vi "Next Identity.vi"(5 "Username":string, 6 "Password":string, 7 "Address":string, 8 "Error In":errorcluster) -> (0 "Error Out":errorcluster)   [LabVIEW 2018, in "Tests.lvlib" / "Agent.lvlib"]
uses:
  Agent.lvlib
  <vilib>/addons/_JKI Toolkits/Caraya/classes/Test/Test.lvclass
  <vilib>/addons/_JKI Toolkits/Caraya/classes/Assert/Assert.lvclass
  src/Toolkit/Agent/Agent.lvclass
  src/Toolkit/Agent Identity/Agent Identity.lvclass
  src/Toolkit/Agent Identity/Support/Create from Agent.vi
  src/Toolkit/Agent/Typedefs/Results.ctl
  src/Toolkit/Agent Identity/Support/Destroy to Agent.vi
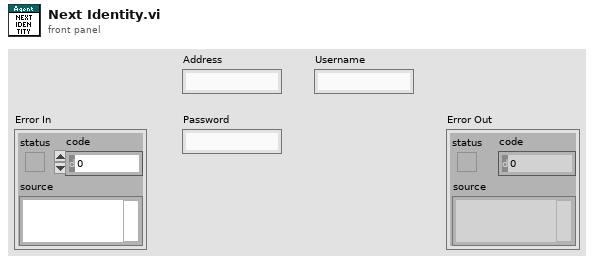
[diagram p1: front panel]
types:
  T1 = typedef "Toolkit.lvlib/Agent.lvclass/Results.ctl" = enum32{"Success", "End of Identities"}
  T2 = typedef "Toolkit.lvlib/Agent.lvclass/Results.ctl" = i32
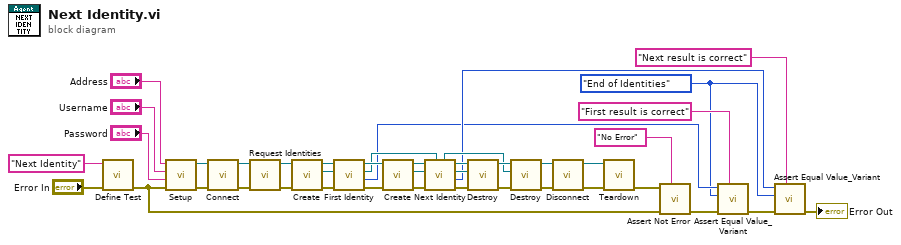
[diagram p0: block diagram]
diagram:
  w1 = Results."End of Identities" ("Result")
  n1 = call <vilib>:"Define Test.vi"("error in (no error)"="Error In", "Label (VI Title)"="Next Identity") -> ("error out"=w36:errorcluster)  [unwired: 9 in]
  n2 = call "Setup.vi"("Error In"=w36, "Password"="Password", "Username"="Username", "Address"="Address") -> ("Error Out"=w34:errorcluster, "Agent"=w35:refnum<class "Agent.lvclass">)  [unwired: 6 in]
  n3 = call "Connect.vi"("Error In"=w34, "Agent In"=w35) -> ("Error Out"=w32:errorcluster, "Agent Out"=w33:refnum<class "Agent.lvclass">)  [unwired: 8 in]
  n4 = call "Request Identities.vi"("Error In"=w32, "Agent In"=w33) -> ("Error Out"=w30:errorcluster, "Agent Out"=w31:refnum<class "Agent.lvclass">)  [unwired: 8 in]
  n5 = call-poly "Create.vi"("Error In"=w30, "Agent In"=w31) -> ("Error Out"=w28:errorcluster, "Identity"=w27:refnum<class "Agent Identity.lvclass">, "Agent Out"=w29:refnum<class "Agent.lvclass">)  [unwired: 7 in]
  n6 = call "First Identity.vi"("Error In"=w28, "Identity In"=w27, "Agent In"=w29) -> ("Error Out"=w17:errorcluster, "Result"=w2:T2, "Identity Out"=w8:refnum<class "Agent Identity.lvclass">, "Agent Out"=w18:refnum<class "Agent.lvclass">)  [unwired: 5 in]
  n7 = call-poly "Create.vi"("Error In"=w17, "Agent In"=w18) -> ("Error Out"=w14:errorcluster, "Identity"=w10:refnum<class "Agent Identity.lvclass">, "Agent Out"=w13:refnum<class "Agent.lvclass">)  [unwired: 7 in]
  n8 = call "Next Identity.vi"("Previous In"=w8, "Error In"=w14, "Next In"=w10, "Agent In"=w13) -> ("Error Out"=w11:errorcluster, "Result"=w6:T2, "Next Out"=w9:refnum<class "Agent Identity.lvclass">, "Agent Out"=w12:refnum<class "Agent.lvclass">, "Previous Out"=w7:refnum<class "Agent Identity.lvclass">)  [unwired: 3 in]
  n9 = call-poly "Destroy.vi"("Error In"=w11, "Identity"=w9, "Agent In"=w12) -> ("Error Out"=w15:errorcluster, "Agent Out"=w16:refnum<class "Agent.lvclass">)  [unwired: 7 in]
  n10 = call-poly "Destroy.vi"("Error In"=w15, "Identity"=w7, "Agent In"=w16) -> ("Error Out"=w24:errorcluster, "Agent Out"=w25:refnum<class "Agent.lvclass">)  [unwired: 7 in]
  n11 = call "Disconnect.vi"("Error In"=w24, "Agent In"=w25) -> ("Error Out"=w23:errorcluster, "Agent Out"=w22:refnum<class "Agent.lvclass">)  [unwired: 8 in]
  n12 = call "Teardown.vi"("Error In"=w23, "Agent"=w22) -> ("Error Out"=w26:errorcluster)  [unwired: 9 in]
  n13 = call <vilib>:"Assert Not Error.vi"("Label"="No Error", "error in (no error)"=w36, "Not Error?"=w26) -> ("error out"=w5:errorcluster)  [unwired: 8 in]
  n14 = call <vilib>:"Assert Equal Value_Variant.vi"("Label"="First result is correct", "error in (no error)"=w5, "Y"=w1, "X"=w2) -> ("error out"=w4:errorcluster)  [unwired: 7 in]
  n15 = call <vilib>:"Assert Equal Value_Variant.vi"("Label"="Next result is correct", "error in (no error)"=w4, "Y"=w1, "X"=w6) -> ("error out"=→"Error Out":errorcluster)  [unwired: 7 in]
